vi "Get All Keys and Values.vi"(8 "error in":errorcluster, 11 "JSON Value in":refnum<class "JSON Value.lvclass">) -> (0 "error out":errorcluster, 1 "values":refnum<class "JSON Value.lvclass">[](array[class]), 2 "keys":string[](array[string]))   [LabVIEW 2016, in "JSON Value.lvclass"]
doc: "Returns an array of all of the keys and an array of their corresponding values. Elements are correlated by index, so the key at a given index corresponds to the value at the same index."
uses:
  JSON Value.lvclass
  JSON Value.lvclass/JSON Value.ctl
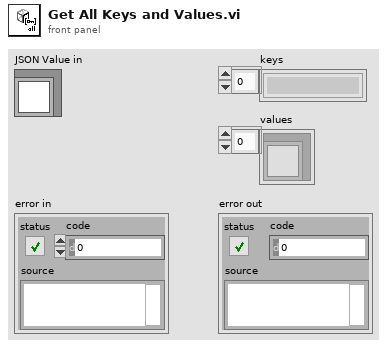
[diagram p1: front panel]
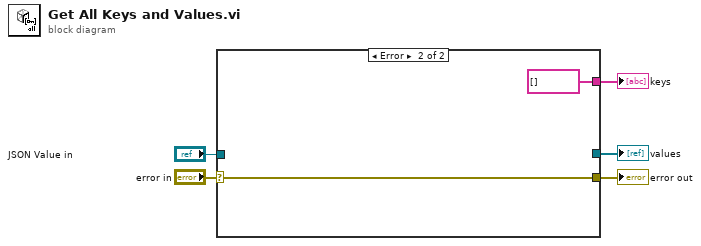
[diagram p0: block diagram]
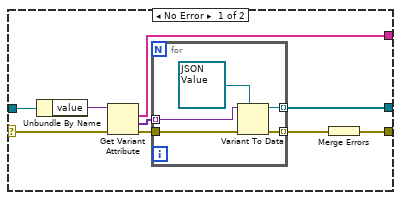
[diagram p2: hidden frame]
diagram:
  n1 = case shown="Error" "error in" {
    selector: "error in" -> [w10 w21]
    tunnel: [w12 string[] []] -> w5
    tunnel: [w11 _] -> w4
    tunnel: [w8 w21] -> w2
    tunnel: "JSON Value in" -> [w9 _]
    frame No Error {
      n2 = Unbundle By Name(w9) -> ("value"=w14:variant)
      n3 = Get Variant Attribute(Variant=w14, error in=w10) -> (names=w12:string[], values=w13:variant[], error out=w6:errorcluster)  [unwired: 2 in, 1 out]
      n4 = for {
        tunnel: w13 -> [w19] mode=indexing
        tunnel: [w18] -> w11 mode=indexing
        tunnel: [w17] -> w7 mode=indexing
        tunnel: w6 -> [w16]
        n5 = Variant To Data(error in=w16, type=refnum<class "JSON Value.lvclass"> refnum ("JSON Object in"), Variant=w19) -> (data=w18:refnum<class "JSON Value.lvclass">, error out=w17:errorcluster)
      }
      n6 = Merge Errors(w7) -> (w8:errorcluster)
    }
    frame Error {
    }
  }
  "keys" <- w5
  "values" <- w4
  "error out" <- w2
